vi "Save Data.vi"(8 "Error In":errorcluster, 10 "Data":string, 11 "reference in":refnum<class "Logger.lvclass">) -> (0 "Error Out":errorcluster, 3 "reference out":refnum<class "Logger.lvclass">)   [LabVIEW 2024, in "Logger.lvclass"]
uses:
  Logger.lvclass
  Logger.lvclass/Logger.ctl
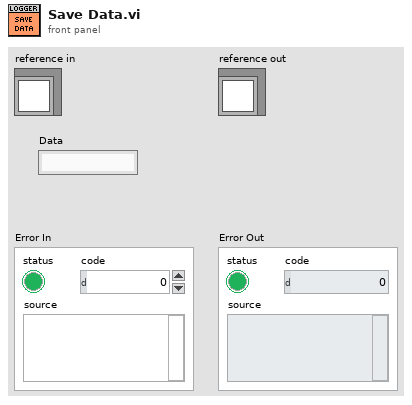
[diagram p1: front panel]
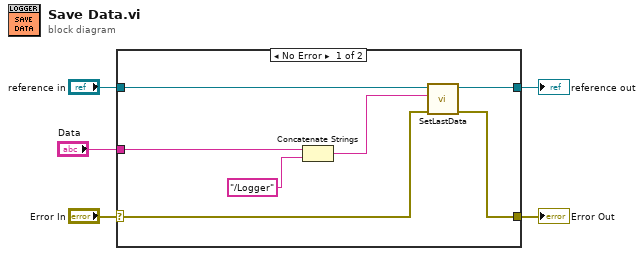
[diagram p0: block diagram]
diagram:
  n1 = case shown="No Error" "Error In" {
    selector: "Error In" -> [w12 w14]
    tunnel: [w9 w14] -> w4
    tunnel: [w7 w13] -> w2
    tunnel: "reference in" -> [w8 w13]
    tunnel: "Data" -> [w11 _]
    frame No Error {
      n2 = Concatenate Strings(w11, "/Logger" ("string")) -> (w6:string)
      n3 = call-dynamic "SetLastData.vi"("Error In"=w12, "LastData"=w6, "reference in"=w8) -> ("Error Out"=w9:errorcluster, "reference out"=w7:refnum<class "Logger.lvclass">)  [unwired: 7 in]
    }
    frame Error {
    }
  }
  "Error Out" <- w4
  "reference out" <- w2
